vi "实验4_3.vi"() -> ()   [LabVIEW 2018]
panel:
  out "XY Graph":cluster{"X":dbl, "Y":dbl}[](graph)
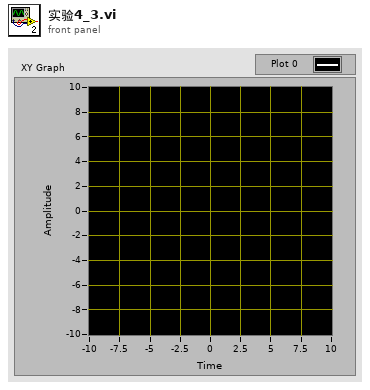
[diagram p1: front panel]
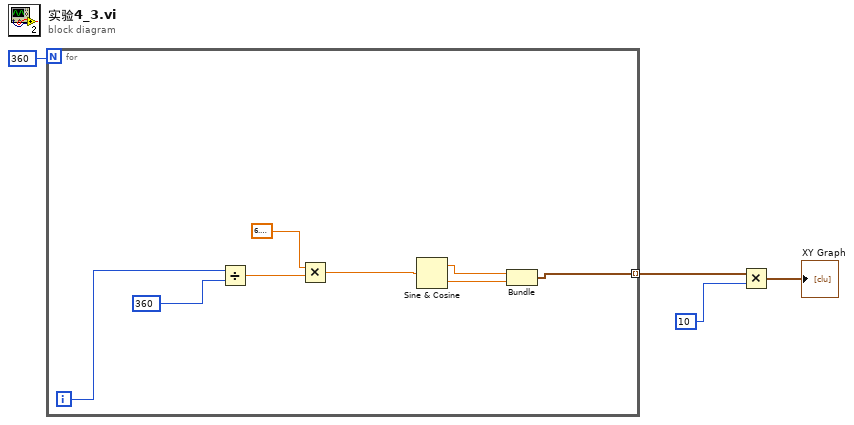
[diagram p0: block diagram]
diagram:
  n1 = for {
    N: 360 -> [_]
    tunnel: [w5] -> w2 mode=indexing
    i -> [w12]
    n2 = Divide(x=w12, y=360) -> (x/y=w10:dbl)
    n3 = Multiply(x=6.283185307179586, y=w10) -> (x*y=w8:dbl)
    n4 = Sine & Cosine(0:w8) -> (1:w7:dbl, 2:w6:dbl)
    n5 = Bundle(w7, w6) -> (w5:cluster{dbl, dbl})  [unwired: 1 in]
  }
  n6 = Multiply(x=w2, y=10) -> (x*y=→"XY Graph":cluster{dbl, dbl}[])
